vi "Open Logging Specification Document.vi"(6 "timeout (ms)":i32=-1, 8 "error in (no error)":errorcluster, 11 "FlexLogger_gRPC in":refnum<class "FlexLogger_gRPC.lvclass">) -> (0 "error out":errorcluster, 1 "document_identifier":T1, 3 "FlexLogger_gRPC out":refnum<class "FlexLogger_gRPC.lvclass">)   [LabVIEW 2020, in "FlexLogger_gRPC.lvlib" / "FlexLogger_gRPC.lvclass"]
uses:
  FlexLogger_gRPC.lvclass
  FlexLogger_client/RPC Messages/flexlogger_ElementIdentifier.ctl
  FlexLogger_client/RPC Messages/flexlogger_OpenLoggingSpecificationDocumentRequest.ctl
  FlexLogger_client/RPC Messages/flexlogger_ProjectIdentifier.ctl
  FlexLogger_gRPC.lvclass/FlexLogger_gRPC.ctl
  FlexLogger_client/FlexLogger_client.lvlib
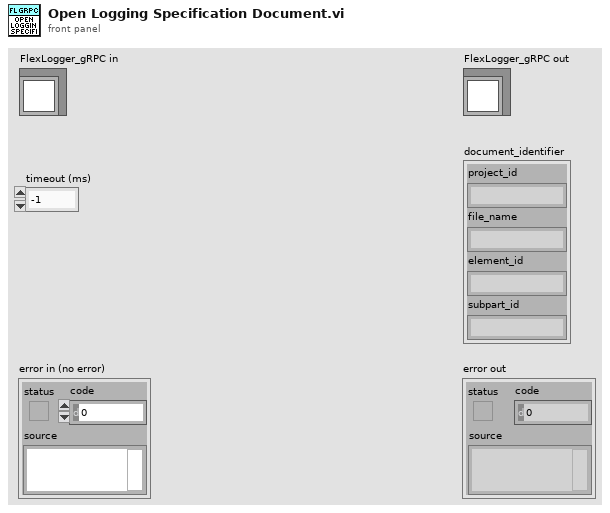
[diagram p1: front panel]
types:
  T1 = typedef "FlexLogger_client.lvlib/flexlogger_ElementIdentifier.ctl" = cluster{"project_id":string, "file_name":string, "element_id":string, "subpart_id":string}
  T2 = typedef "FlexLogger_client.lvlib/flexlogger_OpenLoggingSpecificationDocumentRequest.ctl" = cluster{"project":T3}
  T3 = typedef "FlexLogger_client.lvlib/flexlogger_ProjectIdentifier.ctl" = cluster{"project_id":string}
  T4 = typedef "grpc-lvsupport-release.lvlib/grpcId.ctl" = u64
  T5 = typedef "FlexLogger_client.lvlib/flexlogger_OpenLoggingSpecificationDocumentResponse.ctl" = cluster{"document_identifier":T1}
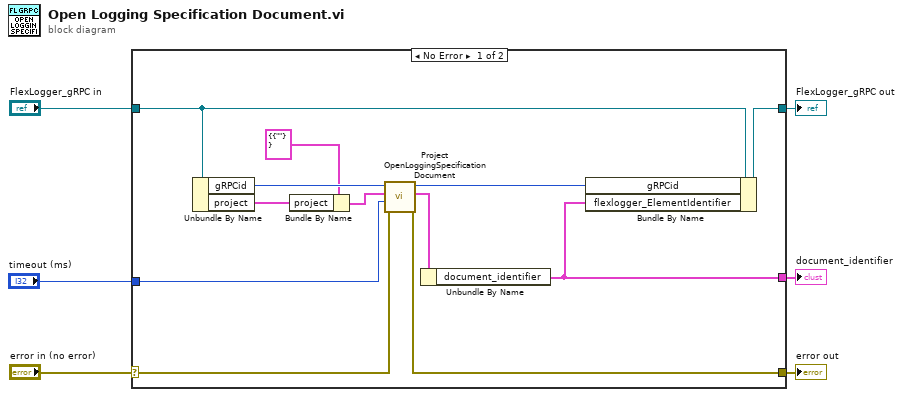
[diagram p0: block diagram]
diagram:
  n1 = case shown="No Error" "error in (no error)" {
    selector: "error in (no error)" -> [w14 w20]
    tunnel: [w13 w20] -> w5
    tunnel: [w17 w19] -> w3
    tunnel: "FlexLogger_gRPC in" -> [w16 w19]
    tunnel: "timeout (ms)" -> [w9 _]
    tunnel: [w7 _] -> w1
    frame No Error {
      n2 = Unbundle By Name(w16) -> ("gRPCid"=w18:T4, "project"=w11:T3)
      n3 = Bundle By Name(cluster=T2 {"project"={"project_id"=""}} ("Request Data"), "project"=w11) -> (w10:T2)
      n4 = call "Project OpenLoggingSpecificationDocument.vi"("error in"=w14, "timeout (ms)"=w9, "Request Data"=w10, "gRPC ID"=w18) -> ("error out"=w13:errorcluster, "Response Data"=w8:T5, "gRPC ID out"=w15:T4)  [unwired: 5 in]
      n5 = Unbundle By Name(w8) -> ("document_identifier"=w7:T1)
      n6 = Bundle By Name(cluster=w16, "gRPCid"=w15, "flexlogger_ElementIdentifier"=w7) -> (w17:refnum<class "FlexLogger_gRPC.lvclass">)
    }
    frame Error {
    }
  }
  "error out" <- w5
  "FlexLogger_gRPC out" <- w3
  "document_identifier" <- w1
